vi "To BananaLeaf.TestSuite.vi"(10 "Properties.Suite":refnum<class "Properties.Suite.lvclass">) -> (3 "Leaf.Properties.TestSuite out":refnum<class "Leaf.Properties.Suite.lvclass">)   [LabVIEW 2021, in "Banana.Caraya.lvlib" / "Leaf.Properties.Suite.lvclass"]
uses:
  Leaf.Properties.Suite.lvclass
  C:/Repositories/LVOS/Bananas/lv-src/Banana.Caraya/Leaf.Properties/Leaf.Properties.lvclass
  <vilib>/addons/_JKI Toolkits/Caraya/classes/Properties.Suite/Properties.Suite.lvclass
  C:/Program Files (x86)/National Instruments/LabVIEW 2021/vi.lib/addons/_JKI Toolkits/Caraya/classes/Properties/Properties.lvclass
  Leaf.Properties/Leaf.Properties.lvclass/Leaf.Properties.ctl
  Leaf.Properties.Suite.lvclass/Leaf.Properties.Suite.ctl
  Leaf.Properties/Leaf.Properties.lvclass
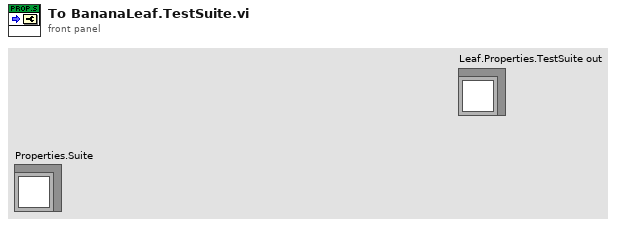
[diagram p1: front panel]
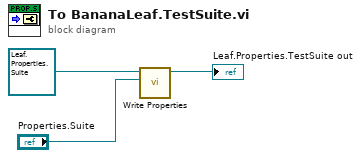
[diagram p0: block diagram]
diagram:
  n1 = call "Write Properties.vi"("Properties"="Properties.Suite", "Leaf.Properties in"=refnum<class "Leaf.Properties.Suite.lvclass"> refnum ("Leaf.Properties.Assert in")) -> ("Leaf.Properties out"=→"Leaf.Properties.TestSuite out":refnum<class "Leaf.Properties.Suite.lvclass">)  [unwired: 9 in]
